vi "仪器电源管理.vi"() -> ()   [LabVIEW 2016, in "环境动力监测库.lvlib" / "V电源管理库.lvlib"]
uses:
  <vilib>/Utility/miscctls.llb/LVPointTypeDef.ctl
  <vilib>/ptbypt/NI_PtbyPt.lvlib
panel:
  in  "主屏看门狗启用":u16(ring) items=["关闭", "打开"]
  in  "主屏看门狗设置":i16
  out "主屏看门狗计时":i16
  in  "照明":bool
  in  "灯带":bool
  in  "R115":i16 caption="灯带关闭时间"
  in  "R114":i16 caption="灯带开启时间"
  in  "电源控制":T1
  # "仪器电源管理"
  # "s"
  # "s"
  # "H"
  # "H"
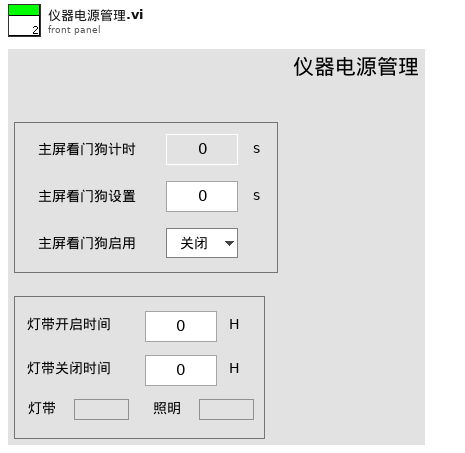
[diagram p1: front panel]
types:
  T1 = cluster{"氨氮电源":bool, "总磷电源":bool, "总氮电源":bool, "多参数电源":bool, "CODMn电源":bool, "CODCr电源":bool}
  T2 = typedef "LVPointTypeDef.ctl" = cluster{"Horizontal":i16, "Vertical":i16}
  T3 = cluster{"状态":cluster{"R0":i16, "R1":i16, "R2":i16, "R3":i16, "R4":i16, "R5":i16, "R6":i16, "R7":i16, "R8":i16, "R9":i16, "R10":i16, "R11":i16, "R12":i16, "R13":i16, "R14":i16, "R15":i16, "R16":i16, "R17":i16, "R18":i16, "R19":i16, "R20":i16, "R21":i16, "R22":i16, "R23":i16, "R24":i16, "R25":i16, "R26":i16, "R27":i16, "R28":i16, "R29":i16, "R30":i16, "R31":i16, "R32":i16, "R33":i16, "R34":i16, "R35":i16, "R36":i16, "R37":i16, "R38":i16, "R39":i16, "R40":i16, "R41":i16, "R42":i16, "R43":i16, "R44":i16, "R45":i16, "R46":i16, "R47":i16, "R48":i16, "R49":i16, "R50":i16, "R51":i16, "R52":i16, "R53":i16, "R54":i16, "R55":i16, "R56":i16, "R57":i16, "R58":i16, "R59":i16, "R60":i16, "R61":i16, "R62":i16, "R63":i16, "R64":i16, "R65":i16, "R66":i16, "R67":i16, "R68":i16, "R69":i16}, "输入状态":bool[], "输出状态":bool[], "报警簇":bool[], "参数设置":cluster{"R100":i16, "R101":i16, "R102":i16, "R103":i16, "R104":i16, "R105":i16, "R106":i16, "R107":i16, "R108":i16, "R109":i16, "R110":i16, "R111":i16, "R112":i16, "R113":i16, "R114":i16, "R115":i16, "R116":i16, "R117":i16, "R118":i16, "R119":i16, "R120":i16, "R121":i16, "R122":i16, "R123":i16, "R124":i16}, "转换值":cluster{"AD0":sgl, "AD1":sgl, "AD2":sgl, "AD3":sgl, "AD4":sgl, "AD5":sgl}, "看门狗启用":bool, "氨氮模块名称":string, "总磷模块名称":string, "采配水模块类型":enum16{"V1", "V2", "V3", "V4", "室内V1", "室内V2"}}
  T4 = cluster{"采配水启用":bool, "CODMn启用":bool, "CODcr启用":bool, "氨氮启用":bool, "总磷启用":bool, "质控单元启用":bool, "流量计启用":bool, "电源管理启用":bool, "其他启用":bool, "多参数启用":bool, "超标留样启用":bool, "总氮启用":bool, "运行模式":enum16{"维护模式", "常规模式", "应急模式", "质控模式"}}
  T5 = cluster{"R0":i16, "R1":i16, "R2":i16, "R3":i16, "R4":i16, "R5":i16, "R6":i16, "R7":i16, "R8":i16, "R9":i16, "R10":i16, "R11":i16, "R12":i16, "R13":i16, "R14":i16, "R15":i16, "R16":i16, "R17":i16, "R18":i16, "R19":i16, "R20":i16, "R21":i16, "R22":i16, "R23":i16, "R24":i16, "R25":i16, "R26":i16, "R27":i16, "R28":i16, "R29":i16, "R30":i16, "R31":i16, "R32":i16, "R33":i16, "R34":i16, "R35":i16, "R36":i16, "R37":i16, "R38":i16, "R39":i16, "R40":i16, "R41":i16, "R42":i16, "R43":i16, "R44":i16, "R45":i16, "R46":i16, "R47":i16, "R48":i16, "R49":i16, "R50":i16, "R51":i16, "R52":i16, "R53":i16, "R54":i16, "R55":i16, "R56":i16, "R57":i16, "R58":i16, "R59":i16, "R60":i16, "R61":i16, "R62":i16, "R63":i16, "R64":i16, "R65":i16, "R66":i16, "R67":i16, "R68":i16, "R69":i16}
  T6 = cluster{"R100":i16, "R101":i16, "R102":i16, "R103":i16, "R104":i16, "R105":i16, "R106":i16, "R107":i16, "R108":i16, "R109":i16, "R110":i16, "R111":i16, "R112":i16, "R113":i16, "R114":i16, "R115":i16, "R116":i16, "R117":i16, "R118":i16, "R119":i16, "R120":i16, "R121":i16, "R122":i16, "R123":i16, "R124":i16}
  T7 = cluster{"网络参数":cluster{"网络状态":bool, "本机IP":string[]}, "电源管理":cluster{"电源管理":bool, "氨氮电源":bool, "总磷电源":bool, "总氮电源":bool, "多参数电源":bool, "CODMn电源":bool, "CODCr电源":bool, "灯带电源":bool, "照明电源":bool}, "北斗-GPS":cluster{"GPS":cluster{"经度:":sgl, "纬度: ":sgl, "GPS监测":bool}, "北斗":cluster{"经度:":sgl, "纬度:":sgl, "北斗监测":bool}}}
  T8 = cluster{"命令":string, "data":cluster{"starting address":u16, "coil values":bool[]}}
  T9 = cluster{"命令":string, "数据":cluster{"starting address":u16, "holding register values":u16[]}}
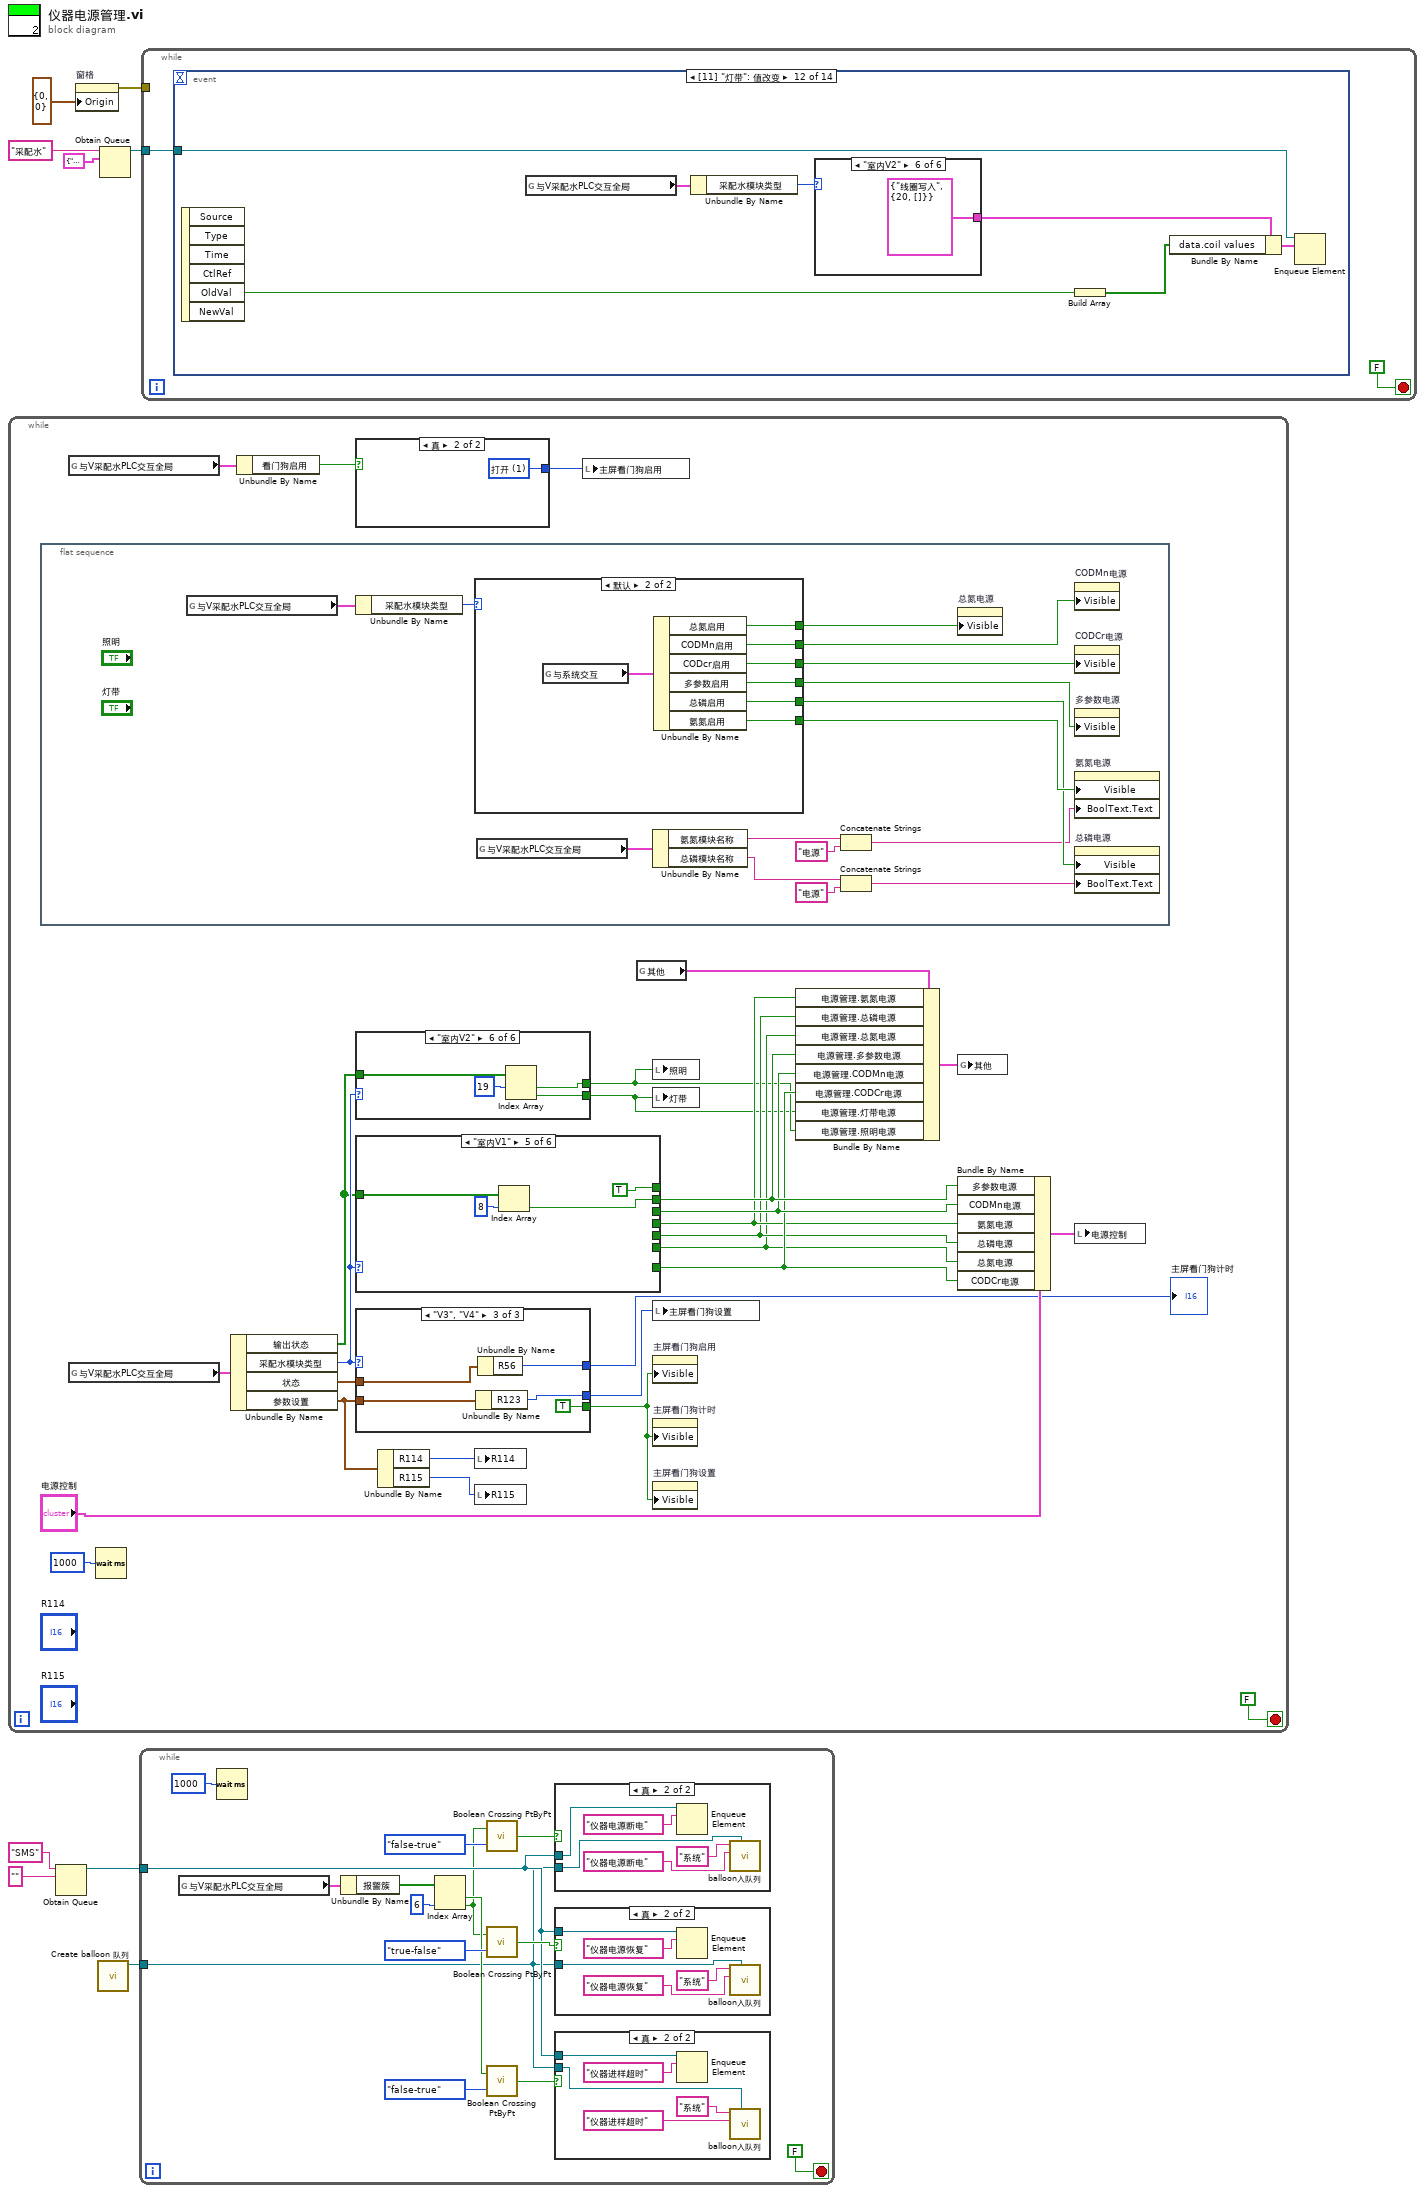
[diagram p0: block diagram]
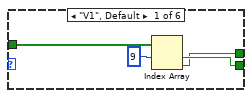
[diagram p5: hidden frame]
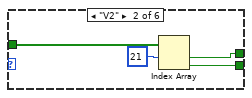
[diagram p6: hidden frame]
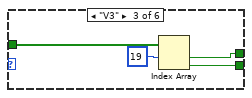
[diagram p7: hidden frame]
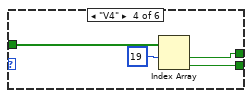
[diagram p8: hidden frame]
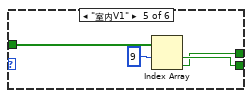
[diagram p9: hidden frame]
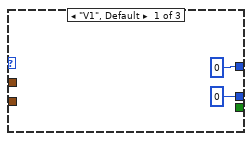
[diagram p10: hidden frame]
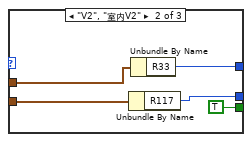
[diagram p11: hidden frame]
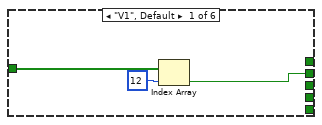
[diagram p12: hidden frame]
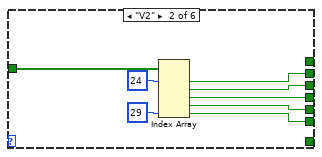
[diagram p13: hidden frame]
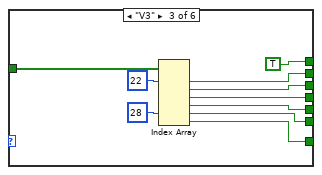
[diagram p14: hidden frame]
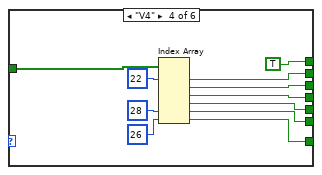
[diagram p15: hidden frame]
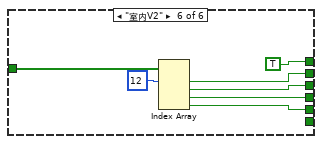
[diagram p16: hidden frame]
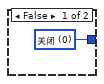
[diagram p17: hidden frame]
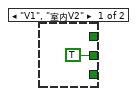
[diagram p18: hidden frame]
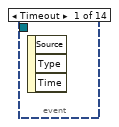
[diagram p19: hidden frame]
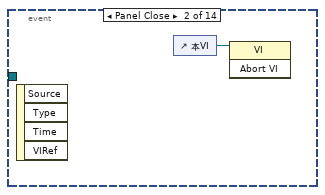
[diagram p20: hidden frame]
diagram:
  n1 = while {
    stop <- FALSE stop-if-true
    n2 = flat-sequence {
      frame #0 {
        n3 = global read "外部交互全局变量.vi" "与V采配水PLC交互全局"() -> (w119:T3)
        n4 = Unbundle By Name(w119) -> ("采配水模块类型"=w118:enum16{"V1", "V2", "V3", "V4", "室内V1", "室内V2"})
        n5 = case shown="默认" w118 {
          tunnel: [_ w139] -> w132
          tunnel: [_ w138] -> w131
          tunnel: [_ w137] -> w130
          tunnel: [_ w136] -> w129
          tunnel: [TRUE ("多参数启用") w135] -> w128
          tunnel: [_ w134] -> w127
          frame "V1", "室内V2" {
          }
          frame Default {
            n6 = global read "外部交互全局变量.vi" "与系统交互"() -> (w140:T4)
            n7 = Unbundle By Name(w140) -> ("总氮启用"=w139:bool, "CODMn启用"=w138:bool, "CODcr启用"=w134:bool, "多参数启用"=w135:bool, "总磷启用"=w136:bool, "氨氮启用"=w137:bool)
          }
        }
        n8 = global read "外部交互全局变量.vi" "与V采配水PLC交互全局"() -> (w125:T3)
        n9 = Unbundle By Name(w125) -> ("氨氮模块名称"=w124:string, "总磷模块名称"=w121:string)
        n10 = Concatenate Strings(w124, "电源" ("字符串")) -> (w123:string)
        n11 = Concatenate Strings(w121, "电源" ("字符串")) -> (w120:string)
        n12 = property on="总氮电源" class="Bool (严格)"("Visible"=w132) -> ()  [unwired: 2 in, 2 out]
        n13 = property on="CODMn电源" class="Bool (严格)"("Visible"=w131) -> ()  [unwired: 2 in, 2 out]
        n14 = property on="CODCr电源" class="Bool (严格)"("Visible"=w127) -> ()  [unwired: 2 in, 2 out]
        n15 = property on="多参数电源" class="Bool (严格)"("Visible"=w128) -> ()  [unwired: 2 in, 2 out]
        n16 = property on="氨氮电源" class="Bool (严格)"("Visible"=w130, "BoolText.Text"=w123) -> ()  [unwired: 2 in, 2 out]
        n17 = property on="总磷电源" class="Bool (严格)"("Visible"=w129, "BoolText.Text"=w120) -> ()  [unwired: 2 in, 2 out]
      }
    }
    n18 = global read "外部交互全局变量.vi" "与V采配水PLC交互全局"() -> (w34:T3)
    n19 = global read "外部交互全局变量.vi" "与V采配水PLC交互全局"() -> (w21:T3)
    n20 = Wait (ms)(milliseconds to wait=u32 1000 ("等待时间（毫秒）")) -> ()  [unwired: 1 out]
    n21 = Unbundle By Name(w21) -> ("输出状态"=w13:bool[], "采配水模块类型"=w14:enum16{"V1", "V2", "V3", "V4", "室内V1", "室内V2"}, "状态"=w22:T5, "参数设置"=w10:T6)
    n22 = Unbundle By Name(w34) -> ("看门狗启用"=w33:bool)
    n23 = case shown="真" w33 {
      tunnel: [w116 w117] -> w32
      frame False {
        w116 = u16 0 items=["关闭", "打开"] ("主屏看门狗启用")
      }
      frame True {
        w117 = u16 1 items=["关闭", "打开"] ("主屏看门狗启用")
      }
    }
    n24 = case shown="\"室内V2\"" w14 {
      tunnel: w13 -> [w39 w41 w45 w51 w55 w59]
      tunnel: [w38 w42 w46 w49 w54 w57] -> w11
      tunnel: [w37 w43 w47 w50 w53 w58] -> w12
      frame "V1", Default {
        n25 = Index Array(array=w39, index #1=9 ("索引")) -> (element #1=w38:bool, element #2=w37:bool)  [unwired: 1 in]
      }
      frame "V2" {
        n26 = Index Array(array=w41, index #1=21 ("索引")) -> (element #1=w43:bool, element #2=w42:bool)  [unwired: 1 in]
      }
      frame "V3" {
        n27 = Index Array(array=w45, index #1=19 ("索引")) -> (element #1=w47:bool, element #2=w46:bool)  [unwired: 1 in]
      }
      frame "V4" {
        n28 = Index Array(array=w51, index #1=19 ("索引")) -> (element #1=w50:bool, element #2=w49:bool)  [unwired: 1 in]
      }
      frame "室内V1" {
        n29 = Index Array(array=w55, index #1=9 ("索引")) -> (element #1=w54:bool, element #2=w53:bool)  [unwired: 1 in]
      }
      frame "室内V2" {
        n30 = Index Array(array=w59, index #1=19 ("索引")) -> (element #1=w58:bool, element #2=w57:bool)  [unwired: 1 in]
      }
    }
    n31 = case shown="\"室内V1\"" w14 {
      tunnel: w13 -> [w75 w83 w93 w104 w108 w115]
      tunnel: [w74 w81 w91 w102 w106 w113] -> w20
      tunnel: [_ w80 w90 w101 _ w111] -> w19
      tunnel: [_ w79 w89 w100 _ w110] -> w17
      tunnel: [_ w78 w88 w99 _ w109] -> w16
      tunnel: [_ w76 w86 w97 _ _] -> w15
      tunnel: [_ _ w85 w96 _ _] -> w18
      tunnel: [_ _ TRUE TRUE TRUE TRUE] -> _
      frame "V1", Default {
        n32 = Index Array(array=w75, index=12 ("索引")) -> (element=w74:bool)
      }
      frame "V2" {
        n33 = Index Array(array=w83, index #1=24 ("索引"), index #5=29 ("索引")) -> (element #1=w81:bool, element #2=w80:bool, element #3=w79:bool, element #4=w78:bool, element #5=w76:bool)  [unwired: 3 in]
      }
      frame "V3" {
        n34 = Index Array(array=w93, index #1=22 ("索引"), index #5=28 ("索引")) -> (element #1=w91:bool, element #2=w90:bool, element #3=w89:bool, element #4=w88:bool, element #5=w86:bool, element #6=w85:bool)  [unwired: 4 in]
      }
      frame "V4" {
        n35 = Index Array(array=w104, index #1=22 ("索引"), index #5=28 ("索引"), index #6=26 ("索引")) -> (element #1=w102:bool, element #2=w101:bool, element #3=w100:bool, element #4=w99:bool, element #5=w97:bool, element #6=w96:bool)  [unwired: 3 in]
      }
      frame "室内V1" {
        n36 = Index Array(array=w108, index=8 ("索引")) -> (element=w106:bool)
      }
      frame "室内V2" {
        n37 = Index Array(array=w115, index #1=12 ("索引")) -> (element #1=w113:bool, element #2=w111:bool, element #3=w110:bool, element #4=w109:bool)  [unwired: 3 in]
      }
    }
    n38 = case shown="\"V3\", \"V4\"" w14 {
      tunnel: [_ TRUE TRUE] -> w25
      tunnel: w22 -> [_ w67 w71]
      tunnel: [i16 0 ("R56") w66 w70] -> w23
      tunnel: w10 -> [_ w65 w69]
      tunnel: [i16 0 ("R123") w64 w68] -> w24
      frame "V1", Default {
      }
      frame "V2", "室内V2" {
        n39 = Unbundle By Name(w65) -> ("R117"=w64:i16)
        n40 = Unbundle By Name(w67) -> ("R33"=w66:i16)
      }
      frame "V3", "V4" {
        n41 = Unbundle By Name(w69) -> ("R123"=w68:i16)
        n42 = Unbundle By Name(w71) -> ("R56"=w70:i16)
      }
    }
    "主屏看门狗计时" <- w23
    n43 = Unbundle By Name(w10) -> ("R114"=w28:i16, "R115"=w29:i16)
    n44 = local write "R114"(w28) -> ()
    n45 = local write "R115"(w29) -> ()
    n46 = local write "主屏看门狗启用"(w32) -> ()
    n47 = global read "内部交互全局变量.vi" "其他"() -> (w30:T7)
    n48 = local write "照明"(w12) -> ()
    n49 = local write "灯带"(w11) -> ()
    n50 = local write "主屏看门狗设置"(w24) -> ()
    n51 = property on="主屏看门狗启用" class="Ring (严格)"("Visible"=w25) -> ()  [unwired: 2 in, 2 out]
    n52 = property on="主屏看门狗计时" class="DigNum (严格)"("Visible"=w25) -> ()  [unwired: 2 in, 2 out]
    n53 = property on="主屏看门狗设置" class="DigNum (严格)"("Visible"=w25) -> ()  [unwired: 2 in, 2 out]
    n54 = Bundle By Name(cluster=w30, "电源管理.氨氮电源"=w17, "电源管理.总磷电源"=w16, "电源管理.总氮电源"=w15, "电源管理.多参数电源"=w20, "电源管理.CODMn电源"=w19, "电源管理.CODCr电源"=w18, "电源管理.灯带电源"=w11, "电源管理.照明电源"=w12) -> (w31:T7)
    n55 = global write "内部交互全局变量.vi" "其他"(w31) -> ()
    n56 = Bundle By Name(cluster="电源控制", "多参数电源"=w20, "CODMn电源"=w19, "氨氮电源"=w17, "总磷电源"=w16, "总氮电源"=w15, "CODCr电源"=w18) -> (w26:T1)
    n57 = local write "电源控制"(w26) -> ()
  }
  n58 = Obtain Queue(name (unnamed)="SMS" ("名称（未命名）"), element data type="" ("名称（未命名）")) -> (queue out=w2:refnum<queue>)  [unwired: 3 in, 2 out]
  n59 = property on="窗格" class="Pane"("Origin"=T2 {"Horizontal"=0, "Vertical"=0} ("原点")) -> (error out=w6:errorcluster)  [unwired: 2 in, 1 out]
  n60 = call "Create balloon 队列.vi"() -> ("队列输出"=w1:refnum<queue>)  [unwired: 11 in]
  n61 = Obtain Queue(name (unnamed)="采配水" ("名称（未命名）"), element data type=cluster{"命令":string, "数据":variant} {"命令"="", "数据"=variant}) -> (queue out=w5:refnum<queue>)  [unwired: 3 in, 2 out]
  n62 = while {
    tunnel: w2 -> [w149]
    tunnel: w1 -> [w143]
    stop <- FALSE stop-if-true
    n63 = global read "外部交互全局变量.vi" "与V采配水PLC交互全局"() -> (w142:T3)
    n64 = Wait (ms)(milliseconds to wait=u32 1000 ("等待时间（毫秒）")) -> ()  [unwired: 1 out]
    n65 = Unbundle By Name(w142) -> ("报警簇"=w141:bool[])
    n66 = Index Array(array=w141, index #2=6 ("索引")) -> (element #1=w146:bool, element #2=w144:bool)  [unwired: 1 in]
    n67 = call <vilib>:"Boolean Crossing PtByPt.vi"("direction"=enum16{"either", "false-true", "true-false"}."false-true", "input"=w144) -> ("crossing"=w152:bool)  [unwired: 1 in]
    n68 = call <vilib>:"Boolean Crossing PtByPt.vi"("direction"=enum16{"either", "false-true", "true-false"}."true-false", "input"=w144) -> ("crossing"=w150:bool)  [unwired: 1 in]
    n69 = call <vilib>:"Boolean Crossing PtByPt.vi"("direction"=enum16{"either", "false-true", "true-false"}."false-true", "input"=w146) -> ("crossing"=w147:bool)  [unwired: 1 in]
    n70 = case shown="真" w152 {
      tunnel: w149 -> [_ w170]
      tunnel: w143 -> [_ w168]
      frame False {
      }
      frame True {
        n71 = Enqueue Element(queue=w170, element="仪器电源断电" ("元素")) -> ()  [unwired: 2 in, 3 out]
        n72 = call "balloon入队列.vi"("队列"=w168, "故障信息"="仪器电源断电" ("元素"), "参数名称"="系统") -> ()  [unwired: 8 in, 1 out]
      }
    }
    n73 = case shown="真" w150 {
      tunnel: w149 -> [_ w163]
      tunnel: w143 -> [_ w162]
      frame False {
      }
      frame True {
        n74 = Enqueue Element(queue=w163, element="仪器电源恢复" ("元素")) -> ()  [unwired: 2 in, 3 out]
        n75 = call "balloon入队列.vi"("队列"=w162, "故障信息"="仪器电源恢复" ("元素"), "参数名称"="系统") -> ()  [unwired: 8 in, 1 out]
      }
    }
    n76 = case shown="真" w147 {
      tunnel: w149 -> [_ w160]
      tunnel: w143 -> [_ w158]
      frame False {
      }
      frame True {
        n77 = Enqueue Element(queue=w160, element="仪器进样超时" ("元素")) -> ()  [unwired: 2 in, 3 out]
        n78 = call "balloon入队列.vi"("队列"=w158, "故障信息"="仪器进样超时" ("元素"), "参数名称"="系统") -> ()  [unwired: 8 in, 1 out]
      }
    }
  }
  n79 = while {
    tunnel: w5 -> [w172]
    tunnel: w6 -> [_]
    stop <- FALSE stop-if-true
    n80 = event shown="[11] \"灯带\": 值改变" {
      selector: _ -> [_ _ _ _ _ _ _ _ _ _ _ _ _ _]
      dyn-events: _ -> [_ _ _ _ _ _ _ _ _ _ _ _ _ _]
      timeout: _ -> [_ _ _ _ _ _ _ _ _ _ _ _ _ _]
      tunnel: w172 -> [_ _ w176 _ w191 w198 w207 w216 w225 w234 w243 w254 w267 w278]
      event Timeout {
        n81 = event-data() -> ()  [unwired: 1 in, 3 out]
      }
      event Panel Close {
        n82 = event-data() -> ()  [unwired: 1 in, 4 out]
        n83 = control-ref of="本VI"() -> (w173:refnum<vi>)
        n84 = invoke class="VI" method="Abort VI"(reference=w173) -> ()  [unwired: 2 in, 3 out]
      }
      event "主屏看门狗启用": Value Change {
        n85 = event-data() -> ("NewVal"=w175:u16)  [unwired: 1 in, 5 out]
        n86 = case shown="0, 默认" w175 {
          tunnel: [FALSE TRUE] -> w174
          frame 0, Default {
          }
          frame 1 {
          }
        }
        n87 = Build Array(w174) -> (w177:bool[])
        n88 = Bundle By Name(cluster=T8 {"命令"="线圈写入", "data"={"starting address"=2800, "coil values"=[]}} ("元素"), "data.coil values"=w177) -> (w178:T8)
        n89 = Enqueue Element(queue=w176, element=w178) -> ()  [unwired: 2 in, 3 out]
      }
      event "主屏看门狗设置", "R114", "R115": Mouse Down {
        n90 = event-data() -> ("CtlRef"=w182:refnum<vi>)  [unwired: 1 in, 5 out]
        n91 = property class="DigNum (严格)"(reference=w182) -> (reference out=w184:refnum<vi>, "Value"=w185:i16)  [unwired: 1 in, 1 out]
        n92 = call "数字键盘.vi"("OldNumber"=w185) -> ("NewNumber"=w183:sgl)
        n93 = property class="DigNum (严格)"(reference=w184, "Val(Sgnl)"=w183) -> ()  [unwired: 1 in, 2 out]
      }
      event "主屏看门狗设置": Value Change {
        n94 = event-data() -> ("NewVal"=w189:i16)  [unwired: 1 in, 5 out]
        n95 = global read "外部交互全局变量.vi" "与V采配水PLC交互全局"() -> (w188:T3)
        n96 = Unbundle By Name(w188) -> ("采配水模块类型"=w187:enum16{"V1", "V2", "V3", "V4", "室内V1", "室内V2"})
        n97 = case shown="\"V3\", \"V4\"" w187 {
          tunnel: [_ u16 117 ("数据.starting address") u16 123 ("数据.starting address")] -> w186
          frame "V1", Default {
          }
          frame "V2", "室内V2" {
          }
          frame "V3", "V4" {
          }
        }
        n98 = Build Array(w189) -> (w190:i16[])
        n99 = Bundle By Name(cluster=T9 {"命令"="多个写入", "数据"={"starting address"=0, "holding register values"=[]}} ("元素"), "数据.starting address"=w186, "数据.holding register values"=w190) -> (w192:T9)
        n100 = Enqueue Element At Opposite End(queue=w191, element=w192) -> ()  [unwired: 2 in, 3 out]
      }
      event "电源控制.多参数电源": Value Change {
        n101 = event-data() -> ("OldVal"=w197:bool)  [unwired: 1 in, 5 out]
        n102 = case shown="真" w197 {
          tunnel: [TRUE ("T button?") w200] -> w196
          frame False {
          }
          frame True {
            n103 = Two Button Dialog(message="请确认是否关闭电源" ("消息")) -> (T button?=w203:bool)  [unwired: 2 in]
            n104 = Select(t=FALSE, s=w203, f=TRUE ("T button?")) -> (s? t:f=w200:bool)
          }
        }
        n105 = call "多参数电源命令.vi"("通电/断电"=w196, "队列"=w198) -> ()  [unwired: 9 in, 1 out]
      }
      event "电源控制.CODMn电源": Value Change {
        n106 = event-data() -> ("OldVal"=w206:bool)  [unwired: 1 in, 5 out]
        n107 = case shown="假" w206 {
          tunnel: [TRUE ("T button?") w209] -> w205
          frame False {
          }
          frame True {
            n108 = Two Button Dialog(message="请确认是否关闭电源" ("消息")) -> (T button?=w212:bool)  [unwired: 2 in]
            n109 = Select(t=FALSE, s=w212, f=TRUE ("T button?")) -> (s? t:f=w209:bool)
          }
        }
        n110 = call "CODMn电源命令.vi"("通电/断电"=w205, "队列"=w207) -> ()  [unwired: 9 in, 1 out]
      }
      event "电源控制.氨氮电源": Value Change {
        n111 = event-data() -> ("OldVal"=w215:bool)  [unwired: 1 in, 5 out]
        n112 = case shown="假" w215 {
          tunnel: [TRUE ("T button?") w218] -> w214
          frame False {
          }
          frame True {
            n113 = Two Button Dialog(message="请确认是否关闭电源" ("消息")) -> (T button?=w221:bool)  [unwired: 2 in]
            n114 = Select(t=FALSE, s=w221, f=TRUE ("T button?")) -> (s? t:f=w218:bool)
          }
        }
        n115 = call "氨氮电源命令.vi"("通电/断电"=w214, "队列"=w216) -> ()  [unwired: 9 in, 1 out]
      }
      event "电源控制.总磷电源": Value Change {
        n116 = event-data() -> ("OldVal"=w224:bool)  [unwired: 1 in, 5 out]
        n117 = case shown="真" w224 {
          tunnel: [TRUE ("T button?") w227] -> w223
          frame False {
          }
          frame True {
            n118 = Two Button Dialog(message="请确认是否关闭电源" ("消息")) -> (T button?=w230:bool)  [unwired: 2 in]
            n119 = Select(t=FALSE, s=w230, f=TRUE ("T button?")) -> (s? t:f=w227:bool)
          }
        }
        n120 = call "总磷电源命令.vi"("通电/断电"=w223, "队列"=w225) -> ()  [unwired: 9 in, 1 out]
      }
      event "电源控制.CODCr电源": Value Change {
        n121 = event-data() -> ("OldVal"=w233:bool)  [unwired: 1 in, 5 out]
        n122 = case shown="真" w233 {
          tunnel: [TRUE ("T button?") w236] -> w232
          frame False {
          }
          frame True {
            n123 = Two Button Dialog(message="请确认是否关闭电源" ("消息")) -> (T button?=w239:bool)  [unwired: 2 in]
            n124 = Select(t=FALSE, s=w239, f=TRUE ("T button?")) -> (s? t:f=w236:bool)
          }
        }
        n125 = call "CODCr电源命令.vi"("通电/断电"=w232, "队列"=w234) -> ()  [unwired: 9 in, 1 out]
      }
      event "电源控制.总氮电源": Value Change {
        n126 = event-data() -> ("OldVal"=w241:bool)  [unwired: 1 in, 5 out]
        n127 = case shown="真" w241 {
          tunnel: [TRUE ("T button?") w245] -> w242
          frame False {
          }
          frame True {
            n128 = Two Button Dialog(message="请确认是否关闭电源" ("消息")) -> (T button?=w248:bool)  [unwired: 2 in]
            n129 = Select(t=FALSE, s=w248, f=TRUE ("T button?")) -> (s? t:f=w245:bool)
          }
        }
        n130 = call "总氮电源命令.vi"("通电/断电"=w242, "队列"=w243) -> ()  [unwired: 9 in, 1 out]
      }
      event "灯带": Value Change {
        n131 = event-data() -> ("OldVal"=w253:bool)  [unwired: 1 in, 5 out]
        n132 = global read "外部交互全局变量.vi" "与V采配水PLC交互全局"() -> (w252:T3)
        n133 = Unbundle By Name(w252) -> ("采配水模块类型"=w251:enum16{"V1", "V2", "V3", "V4", "室内V1", "室内V2"})
        n134 = case shown="\"室内V2\"" w251 {
          tunnel: [T8 {"命令"="线圈写入", "data"={"starting address"=2451, "coil values"=[]}} ("元素") T8 {"命令"="线圈写入", "data"={"starting address"=2451, "coil values"=[]}} ("元素") T8 {"命令"="线圈写入", "data"={"starting address"=2450, "coil values"=[]}} ("元素") T8 {"命令"="线圈写入", "data"={"starting address"=2450, "coil values"=[]}} ("元素") T8 {"命令"="线圈写入", "data"={"starting address"=9, "coil values"=[]}} ("元素") T8 {"命令"="线圈写入", "data"={"starting address"=20, "coil values"=[]}} ("元素")] -> w250
          frame "V1", Default {
          }
          frame "V2" {
          }
          frame "V3" {
          }
          frame "V4" {
          }
          frame "室内V1" {
          }
          frame "室内V2" {
          }
        }
        n135 = Build Array(w253) -> (w255:bool[])
        n136 = Bundle By Name(cluster=w250, "data.coil values"=w255) -> (w256:T8)
        n137 = Enqueue Element(queue=w254, element=w256) -> ()  [unwired: 2 in, 3 out]
      }
      event "照明": Value Change {
        n138 = event-data() -> ("NewVal"=w266:bool)  [unwired: 1 in, 5 out]
        n139 = global read "外部交互全局变量.vi" "与V采配水PLC交互全局"() -> (w264:T3)
        n140 = Unbundle By Name(w264) -> ("采配水模块类型"=w265:enum16{"V1", "V2", "V3", "V4", "室内V1", "室内V2"})
        n141 = case shown="\"V2\"" w265 {
          tunnel: [T8 {"命令"="线圈写入", "data"={"starting address"=2452, "coil values"=[]}} ("元素") T8 {"命令"="线圈写入", "data"={"starting address"=2452, "coil values"=[]}} ("元素") T8 {"命令"="线圈写入", "data"={"starting address"=2452, "coil values"=[]}} ("元素") T8 {"命令"="线圈写入", "data"={"starting address"=2452, "coil values"=[]}} ("元素") T8 {"命令"="线圈写入", "data"={"starting address"=10, "coil values"=[]}} ("元素") T8 {"命令"="线圈写入", "data"={"starting address"=19, "coil values"=[]}} ("元素")] -> w263
          frame "V1", Default {
          }
          frame "V2" {
          }
          frame "V3" {
          }
          frame "V4" {
          }
          frame "室内V1" {
          }
          frame "室内V2" {
          }
        }
        n142 = Build Array(w266) -> (w268:bool[])
        n143 = Bundle By Name(cluster=w263, "data.coil values"=w268) -> (w269:T8)
        n144 = Enqueue Element(queue=w267, element=w269) -> ()  [unwired: 2 in, 3 out]
      }
      event "R114", "R115": Value Change {
        n145 = event-data() -> ()  [unwired: 1 in, 6 out]
        n146 = local read "R114"() -> (w277:i16)
        n147 = local read "R115"() -> (w276:i16)
        n148 = Build Array(w277, w276) -> (w279:i16[])
        n149 = Bundle By Name(cluster=T9 {"命令"="多个写入", "数据"={"starting address"=0, "holding register values"=[]}} ("元素"), "数据.starting address"=u16 114, "数据.holding register values"=w279) -> (w280:T9)
        n150 = Enqueue Element At Opposite End(queue=w278, element=w280) -> ()  [unwired: 2 in, 3 out]
      }
    }
  }
